vi "Read Output Till Settle.vi"(7 "timeout [ms]":u32=2000, 8 "error in":errorcluster, 10 "settled for [ms]":u32=1000, 11 "GOLPI ref. in":T1={"pipe handle"={"lv_proc.dll file path"=path "", "process instance handle"=[], "debug mode"=FALSE, "debug data"=[]}, "fast read timeout [ms]"=500, "fast read settle time [ms]"=10, "fast read to multiple [ms]"=1, "max elements per input line"=100, "slow read timeout [ms]"=500, "stdin double format specifier"="%_16e", "max elements per stdout output column"=100, "console mode bitstream"=FALSE, "bitstream first read timeout [ms]"=1000, "bitstream read timeout [ms]"=50, "struct transfer possible"=FALSE, "matlab mode"=FALSE}) -> (0 "error out":errorcluster, 2 "read buffer":string, 3 "GOLPI ref. out":T1={"pipe handle"={"lv_proc.dll file path"=path "", "process instance handle"=[], "debug mode"=FALSE, "debug data"=[]}, "fast read timeout [ms]"=500, "fast read settle time [ms]"=10, "fast read to multiple [ms]"=1, "max elements per input line"=100, "slow read timeout [ms]"=500, "stdin double format specifier"="%_16e", "max elements per stdout output column"=100, "console mode bitstream"=FALSE, "bitstream first read timeout [ms]"=1000, "bitstream read timeout [ms]"=50, "struct transfer possible"=FALSE, "matlab mode"=FALSE}, 5 "bytes remaining":i32)   [LabVIEW 2020, in "GOLPI library.lvlib"]
doc: "Continually reads output of GNU Octave. If no new data appears in the buffer for at least 'settled for' miliseconds, reading stops. If timeout is exceeded, returns only part of buffer and returns number of bytes remaining in the stdout (if any).\n\n---\nGOLPI works only with lv_proc.dll library, which is part of vipm package or should be delivered together with packed library. Placement of this dll is selected in terminal of Start GNU Octave.vi."
uses:
  GOLPI library.lvlib
  GOLPI reference Type Def.ctl
  Pipe Handle.ctl
  Custom Error Codes Enum Type Def.vi
  LV Process library.lvlib
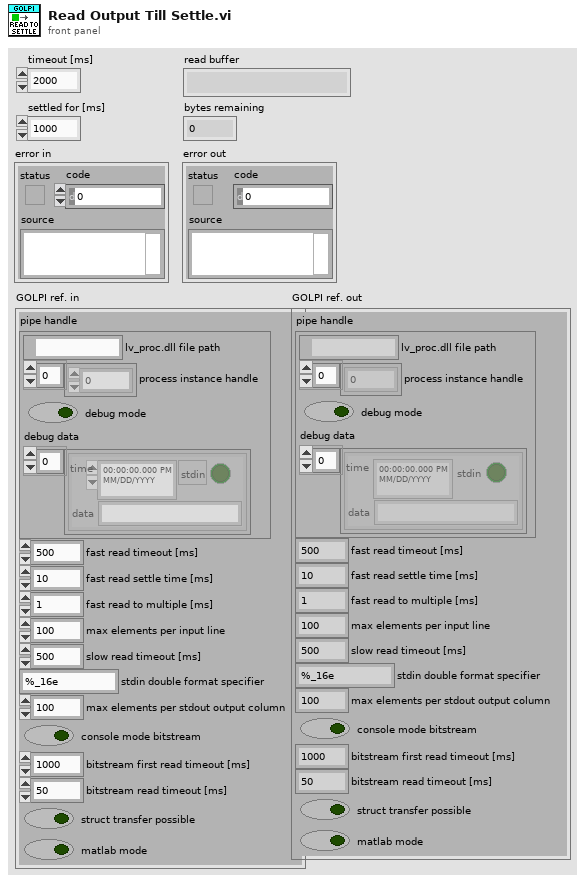
[diagram p1: front panel]
types:
  T1 = typedef "GOLPI library.lvlib/GOLPI reference Type Def.ctl" = cluster{"pipe handle":T2, "fast read timeout [ms]":u32, "fast read settle time [ms]":u32, "fast read to multiple [ms]":u32, "max elements per input line":u32, "slow read timeout [ms]":u32, "stdin double format specifier":string, "max elements per stdout output column":u32, "console mode bitstream":bool, "bitstream first read timeout [ms]":u32, "bitstream read timeout [ms]":u32, "struct transfer possible":bool, "matlab mode":bool}
  T2 = typedef "LV Process library.lvlib/Pipe Handle.ctl" = cluster{"lv_proc.dll file path":path, "process instance handle":u32[], "debug mode":bool, "debug data":cluster{"time":timestamp, "stdin":bool, "data":string}[]}
  T3 = typedef "GOLPI library.lvlib/Custom Error Codes Enum Type Def.vi" = enum16{"no error", "00 working directory PAR1 missing", "01 octave binary PAR1 missing", "02 octave report error PAR1", "03 empty output last cmd PAR1", "04 missing temporary file PAR1", "05 pwd PAR 1 not exist", "06 oct package not installed", "07 octave default binary missing", "10 var PAR1 not string, vect", "11 var PAR1 not num, scal, ~compl", "12 var PAR1 not num, scal, compl", "13 var PAR1 not num, vect, ~compl", "14 var PAR1 not num, vect, compl", "15 var PAR1 not num, mat, ~compl", "16 var PAR1 not num, mat, ~compl", "30 read timeout", "60 bitstream transport failed", "61 bitstream decode error PAR1", "62 bitstream cannot be set", "70 struct transfer not possible", "80 struct: cluster elem. PAR1 not implem.", "81 struct: structure field PAR1 not implem.", "82 struct: size mismatch of PAR1", "83 struct: type mismatch of PAR1", "98 internal error", "99 not finished", "90 Not supported in Matlab mode", "91 Matlab variable transfer error", "92 Matlab Script Error"}
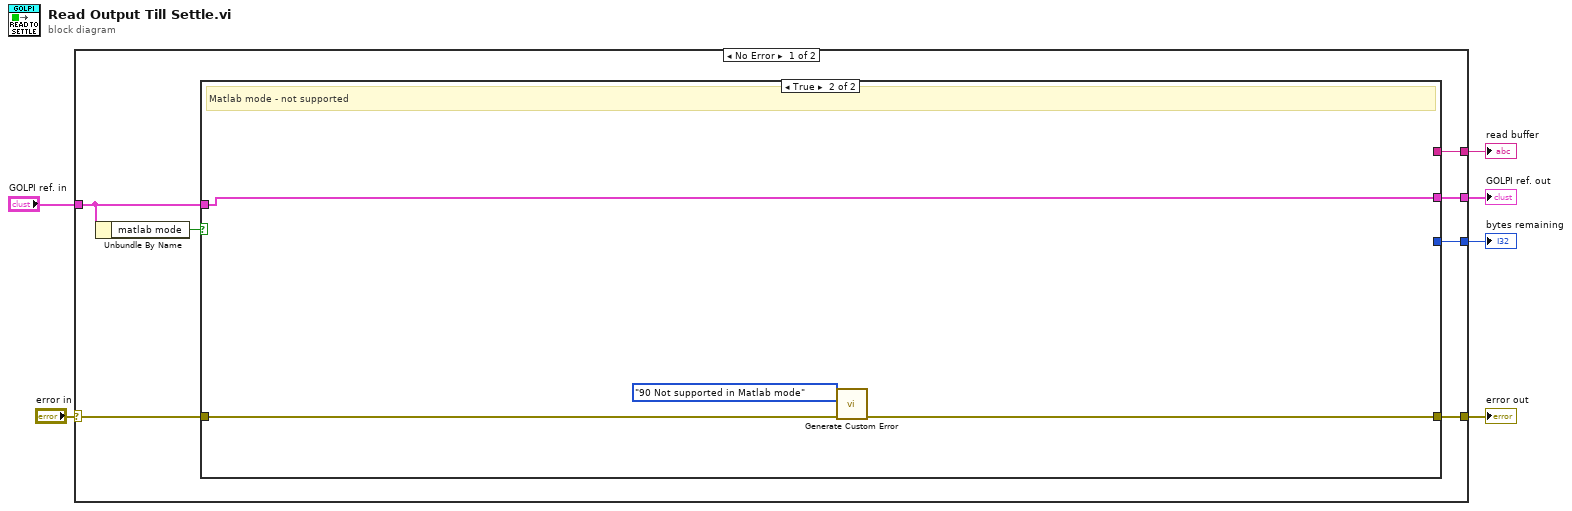
[diagram p0: block diagram]
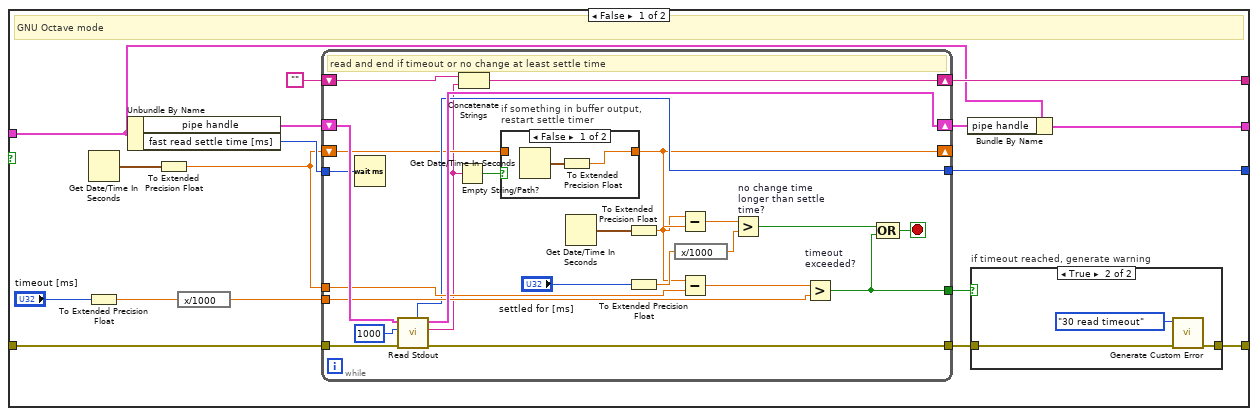
[diagram p2: hidden frame]
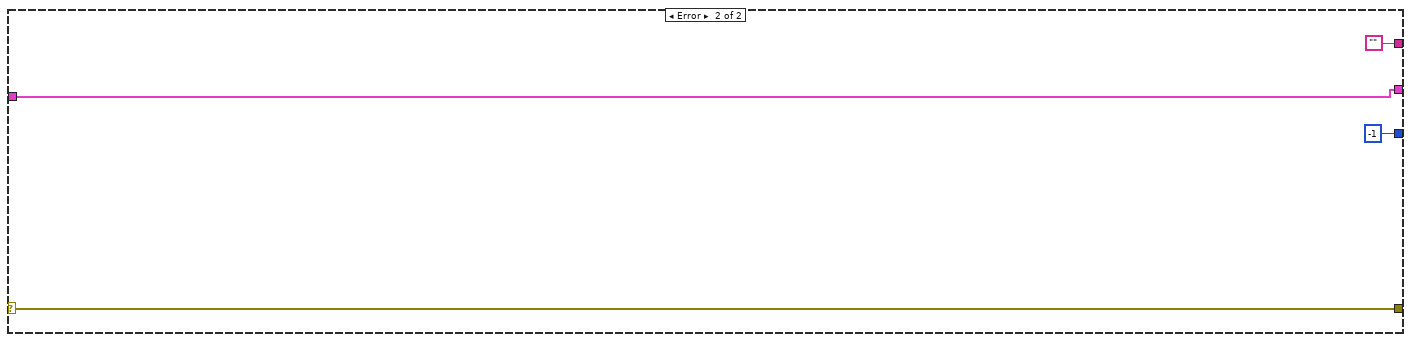
[diagram p5: hidden frame]
diagram:
  n1 = case shown="No Error" "error in" {
    selector: "error in" -> [w9 w70]
    tunnel: [w13 ""] -> w6
    tunnel: [w12 -1 ("bytes remaining")] -> w5
    tunnel: [w11 w67] -> w4
    tunnel: "GOLPI ref. in" -> [w8 w67]
    tunnel: [w10 w70] -> w2
    frame No Error {
      n2 = Unbundle By Name(w8) -> ("matlab mode"=w7:bool)
      n3 = case shown="True" w7 {
        tunnel: [w30 _] -> w13
        tunnel: [w29 _] -> w12
        tunnel: [w26 w64] -> w11
        tunnel: w8 -> [w25 w64]
        tunnel: [w20 w65] -> w10
        tunnel: w9 -> [w19 w66]
        frame False {
          # "GNU Octave mode"
          n4 = Get Date/Time In Seconds() -> (seconds since 1Jan1904=w15:timestamp)
          n5 = To Extended Precision Float(1:"timeout [ms]") -> (0:w17:ext)
          n6 = Unbundle By Name(w25) -> ("pipe handle"=w27:T2, "fast read settle time [ms]"=w23:u32)
          n7 = To Extended Precision Float(1:w15) -> (0:w14:ext)
          n8 = expression code="x/1000"(w17) -> (w16:ext)
          n9 = while {
            tunnel: [w57] -> w21
            tunnel: w19 -> [w56]
            tunnel: [w51] -> w29
            shift-right: [w58] -> w24
            shift-left: w27 -> [w59]
            shift-right: [w55] -> w30
            shift-left: "" -> [w48]
            tunnel: w14 -> [w54]
            tunnel: w16 -> [w52]
            shift-right: [w43] -> _
            shift-left: w14 -> [w47]
            tunnel: w23 -> [w41]
            tunnel: [w40] -> w22
            stop <- w50 stop-if-true
            # "read and end if timeout or no change at least settle time"
            n10 = Wait (ms)(milliseconds to wait=w41) -> ()  [unwired: 1 out]
            n11 = call "Read Stdout.vi"("error in"=w56, "byte count"=1000, "pipe in"=w59) -> ("error out"=w57:errorcluster, "read buffer"=w44:string, "pipe out"=w58:T2, "bytes remaining"=w51:i32)  [unwired: 3 in, 2 out]
            n12 = Empty String/Path?(string/path=w44) -> (empty?=w45:bool)
            n13 = Concatenate Strings(w48, w44) -> (w55:string)
            n14 = case "if something in buffer output,\nrestart settle timer" shown="False" w45 {
              tunnel: [w60 w62] -> w43
              tunnel: w47 -> [_ w62]
              frame False {
                n15 = Get Date/Time In Seconds() -> (seconds since 1Jan1904=w61:timestamp)
                n16 = To Extended Precision Float(1:w61) -> (0:w60:ext)
              }
              frame True {
              }
            }
            n17 = Get Date/Time In Seconds() -> (seconds since 1Jan1904=w36:timestamp)
            n18 = To Extended Precision Float(1:w36) -> (0:w35:ext)
            n19 = To Extended Precision Float(1:"settled for [ms]") -> (0:w39:ext)
            n20 = expression code="x/1000"(w39) -> (w37:ext)
            n21 = Subtract(x=w35, y=w43) -> (x-y=w42:ext)
            n22 = Subtract(x=w35, y=w54) -> (x-y=w53:ext)
            n23 = Greater? "no change time\nlonger than settle\ntime?"(x=w42, y=w37) -> (0:w46:bool)
            n24 = Greater? "timeout\nexceeded?"(x=w53, y=w52) -> (0:w40:bool)
            n25 = Compound Arithmetic op=OR(w46, w40) -> (w50:bool)
          }
          n26 = Bundle By Name(cluster=w25, "pipe handle"=w24) -> (w26:T1)
          n27 = case "if timeout reached, generate warning" shown="True" w22 {
            tunnel: [w31 w32] -> w20
            tunnel: w21 -> [w31 w33]
            frame False {
            }
            frame True {
              n28 = call "Generate Custom Error.vi"("error in"=w33, "GOLPI error"=Custom_Error_Codes_Enum_Type_Def.vi."30 read timeout") -> ("error out"=w32:errorcluster)  [unwired: 9 in]
            }
          }
        }
        frame True {
          # "Matlab mode - not supported"
          n29 = call "Generate Custom Error.vi"("error in"=w66, "GOLPI error"=Custom_Error_Codes_Enum_Type_Def.vi."90 Not supported in Matlab mode") -> ("error out"=w65:errorcluster)  [unwired: 9 in]
        }
      }
    }
    frame Error {
    }
  }
  "error out" <- w2
  "read buffer" <- w6
  "bytes remaining" <- w5
  "GOLPI ref. out" <- w4
